vi "StepperMain.vi"() -> ()   [LabVIEW 2014]
uses:
  <vilib>/Instr/_visa.llb/VISA Configure Serial Port (Instr).vi
panel:
  in  "Jump":string caption="String"
  in  "Move":string caption="String"
  in  "Interleaved?":bool
  in  "Jump Button":bool
  in  "Step forward":bool
  in  "Step backward":bool
  in  "+1":bool
  in  "-1":bool
  in  "Home Button":bool
  in  "stop":bool
  out "Position":string
  in  "Com Port":refnum<visa-resource-name>
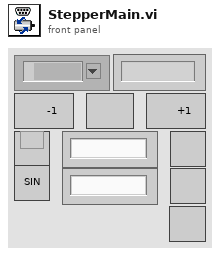
[diagram p1: front panel]
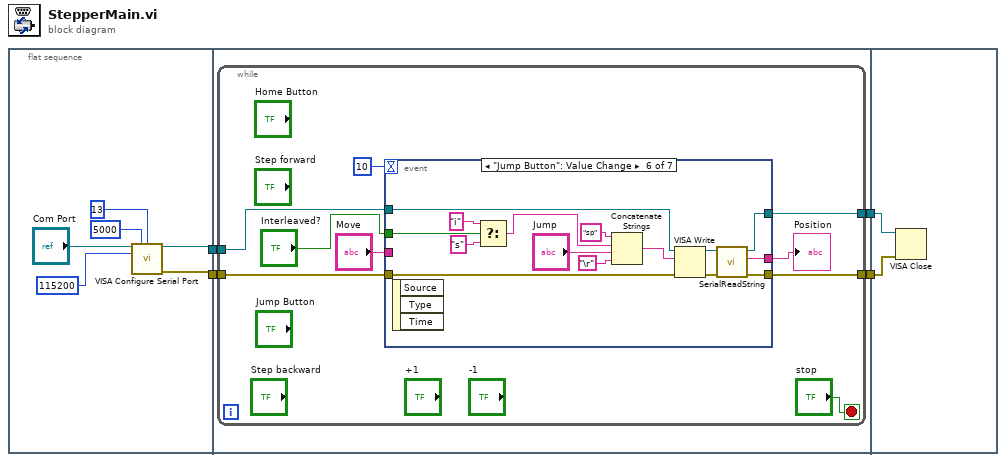
[diagram p0: block diagram]
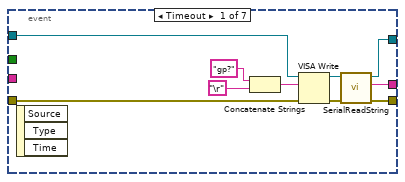
[diagram p2: hidden frame]
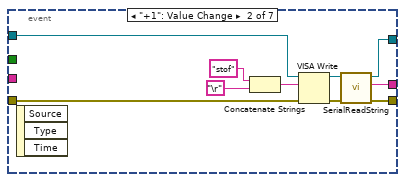
[diagram p3: hidden frame]
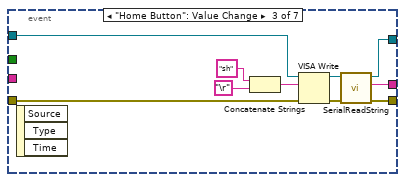
[diagram p4: hidden frame]
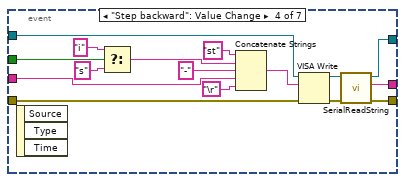
[diagram p5: hidden frame]
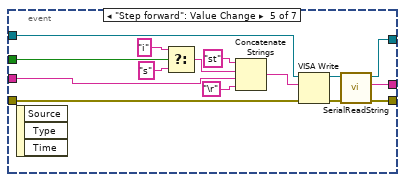
[diagram p6: hidden frame]
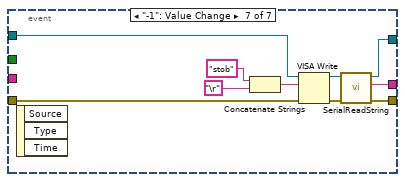
[diagram p7: hidden frame]
diagram:
  n1 = flat-sequence {
    tunnel: [w6] -> w2
    tunnel: [w5] -> w1
    tunnel: [w12] -> w4
    tunnel: [w11] -> w3
    tunnel: w2 -> [w14]
    tunnel: w1 -> [w13]
    tunnel: w4 -> [w111]
    tunnel: w3 -> [w110]
    frame #0 {
      n2 = call-poly "VISA Configure Serial Port"("VISA resource name"="Com Port", "timeout (10sec)"=u32 5000, "termination char\n(0xA = '\\n' = LF)"=u8 13 ("termination char\n(0xA = '\\n' = LF)"), "baud rate (9600)"=u32 115200) -> ("VISA resource name out"=w6:refnum<visa-resource-name>, "error out"=w5:errorcluster)  [unwired: 10 in]
    }
    frame #1 {
      n3 = while {
        tunnel: w14 -> [w22]
        tunnel: w13 -> [w21]
        tunnel: [w20] -> w11
        tunnel: [w19] -> w12
        stop <- "stop" stop-if-true
        n4 = event shown="[5] \"Jump Button\": Value Change" {
          selector: _ -> [_ _ _ _ _ _ _]
          dyn-events: _ -> [_ _ _ _ _ _ _]
          timeout: 10 -> [_ _ _ _ _ _ _]
          tunnel: w22 -> [w33 w42 w51 w63 w77 w91 w107]
          tunnel: w21 -> [w32 w43 w50 w64 w75 w87 w106]
          tunnel: [w29 w40 w48 w65 w72 w88 w104] -> w20
          tunnel: [w30 w41 w49 w67 w74 w90 w105] -> w19
          tunnel: [w28 w37 w47 w66 w73 w89 w103] -> w17
          tunnel: "Interleaved?" -> [_ _ _ w62 w76 w92 _]
          tunnel: "Move" -> [_ _ _ w55 w71 _ _]
          event Timeout {
            n5 = event-data() -> ()  [unwired: 1 in, 3 out]
            n6 = Concatenate Strings("gp?" ("write buffer"), "\r") -> (w26:string)
            n7 = VISA Write(VISA resource name=w33, write buffer=w26, error in (no error)=w32) -> (VISA resource name out=w31:refnum<visa-resource-name>, error out=w27:errorcluster)  [unwired: 1 out]
            n8 = call "SerialReadString.vi"("error in (no error)"=w27, "VISA Refnum in"=w31) -> ("error out"=w29:errorcluster, "trimmed string"=w28:string, "VISA Refnum out"=w30:refnum<visa-resource-name>)  [unwired: 7 in]
          }
          event "+1": Value Change {
            n9 = event-data() -> ()  [unwired: 1 in, 3 out]
            n10 = Concatenate Strings("stof" ("write buffer"), "\r") -> (w35:string)
            n11 = VISA Write(VISA resource name=w42, write buffer=w35, error in (no error)=w43) -> (VISA resource name out=w39:refnum<visa-resource-name>, error out=w38:errorcluster)  [unwired: 1 out]
            n12 = call "SerialReadString.vi"("error in (no error)"=w38, "VISA Refnum in"=w39) -> ("error out"=w40:errorcluster, "trimmed string"=w37:string, "VISA Refnum out"=w41:refnum<visa-resource-name>)  [unwired: 7 in]
          }
          event "Home Button": Value Change {
            n13 = event-data() -> ()  [unwired: 1 in, 3 out]
            n14 = Concatenate Strings("sh" ("write buffer"), "\r") -> (w45:string)
            n15 = VISA Write(VISA resource name=w51, write buffer=w45, error in (no error)=w50) -> (VISA resource name out=w52:refnum<visa-resource-name>, error out=w53:errorcluster)  [unwired: 1 out]
            n16 = call "SerialReadString.vi"("error in (no error)"=w53, "VISA Refnum in"=w52) -> ("error out"=w48:errorcluster, "trimmed string"=w47:string, "VISA Refnum out"=w49:refnum<visa-resource-name>)  [unwired: 7 in]
          }
          event "Step backward": Value Change {
            n17 = event-data() -> ()  [unwired: 1 in, 3 out]
            n18 = Select(t="i", s=w62, f="s") -> (s? t:f=w58:string)
            n19 = Concatenate Strings("st", w58, "-" ("string"), w55, "\r") -> (w57:string)
            n20 = VISA Write(VISA resource name=w63, write buffer=w57, error in (no error)=w64) -> (VISA resource name out=w69:refnum<visa-resource-name>, error out=w68:errorcluster)  [unwired: 1 out]
            n21 = call "SerialReadString.vi"("error in (no error)"=w68, "VISA Refnum in"=w69) -> ("error out"=w65:errorcluster, "trimmed string"=w66:string, "VISA Refnum out"=w67:refnum<visa-resource-name>)  [unwired: 7 in]
          }
          event "Step forward": Value Change {
            n22 = event-data() -> ()  [unwired: 1 in, 3 out]
            n23 = Select(t="i", s=w76, f="s") -> (s? t:f=w83:string)
            n24 = Concatenate Strings("st", w83, w71, "\r") -> (w84:string)
            n25 = VISA Write(VISA resource name=w77, write buffer=w84, error in (no error)=w75) -> (VISA resource name out=w78:refnum<visa-resource-name>, error out=w79:errorcluster)  [unwired: 1 out]
            n26 = call "SerialReadString.vi"("error in (no error)"=w79, "VISA Refnum in"=w78) -> ("error out"=w72:errorcluster, "trimmed string"=w73:string, "VISA Refnum out"=w74:refnum<visa-resource-name>)  [unwired: 7 in]
          }
          event "Jump Button": Value Change {
            n27 = event-data() -> ()  [unwired: 1 in, 3 out]
            n28 = Select(t="i", s=w92, f="s") -> (s? t:f=w94:string)
            n29 = Concatenate Strings("sp", w94, "Jump", "\r") -> (w93:string)
            n30 = VISA Write(VISA resource name=w91, write buffer=w93, error in (no error)=w87) -> (VISA resource name out=w99:refnum<visa-resource-name>, error out=w98:errorcluster)  [unwired: 1 out]
            n31 = call "SerialReadString.vi"("error in (no error)"=w98, "VISA Refnum in"=w99) -> ("error out"=w88:errorcluster, "trimmed string"=w89:string, "VISA Refnum out"=w90:refnum<visa-resource-name>)  [unwired: 7 in]
          }
          event "-1": Value Change {
            n32 = event-data() -> ()  [unwired: 1 in, 3 out]
            n33 = Concatenate Strings("stob" ("write buffer"), "\r") -> (w100:string)
            n34 = VISA Write(VISA resource name=w107, write buffer=w100, error in (no error)=w106) -> (VISA resource name out=w108:refnum<visa-resource-name>, error out=w109:errorcluster)  [unwired: 1 out]
            n35 = call "SerialReadString.vi"("error in (no error)"=w109, "VISA Refnum in"=w108) -> ("error out"=w104:errorcluster, "trimmed string"=w103:string, "VISA Refnum out"=w105:refnum<visa-resource-name>)  [unwired: 7 in]
          }
        }
        "Position" <- w17
      }
    }
    frame #2 {
      n36 = VISA Close(VISA resource name=w111, error in (no error)=w110) -> ()  [unwired: 1 out]
    }
  }
